vi "Mask from ROI.vi"(6 "Shrink":bool, 7 "ROI Descriptor":T1 {"Contours"."Type" items=["No Selection", "Point", "Line", "Rectangle", "Oval", "Polygon", "Free", "Annulus", "Unused2", "Unused3", "Broken Line", "Free Hand Line", "Rotated Rectangle"]}, 8 "error in (no error)":errorcluster, 9 "Out / In":bool, 11 "Image Src":T2) -> (0 "error out":errorcluster, 3 "Image Out":T2)   [LabVIEW 2014]
doc: "Recopies the Image Src into the Image Dst. You can specify if the pixels that are inside the ROI or outside the ROI are set to 0."
uses:
  <vilib>/vision/Image Controls.llb/IMAQ Image.ctl
  <vilib>/vision/NI_Vision_Development_Module.lvlib
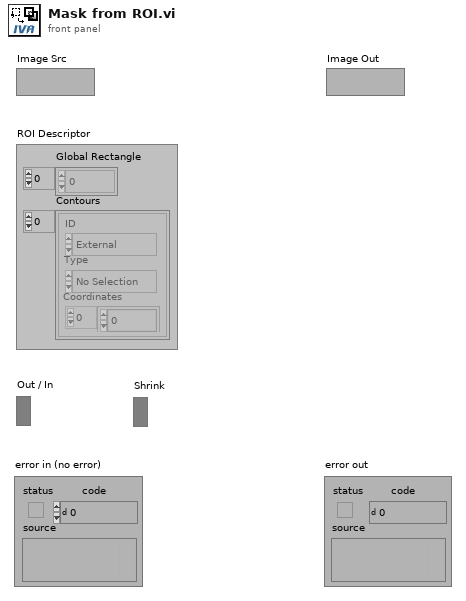
[diagram p1: front panel]
types:
  T1 = cluster{"Global Rectangle":i32[], "Contours":cluster{"ID":enum32{"External", "Internal"}, "Type":u32, "Coordinates":i32[]}[]}
  T2 = typedef "IMAQ Image.ctl" = refnum<image>
  T3 = cluster{"ID":enum32{"External", "Internal"}, "Type":u32, "Coordinates":i32[]}[]
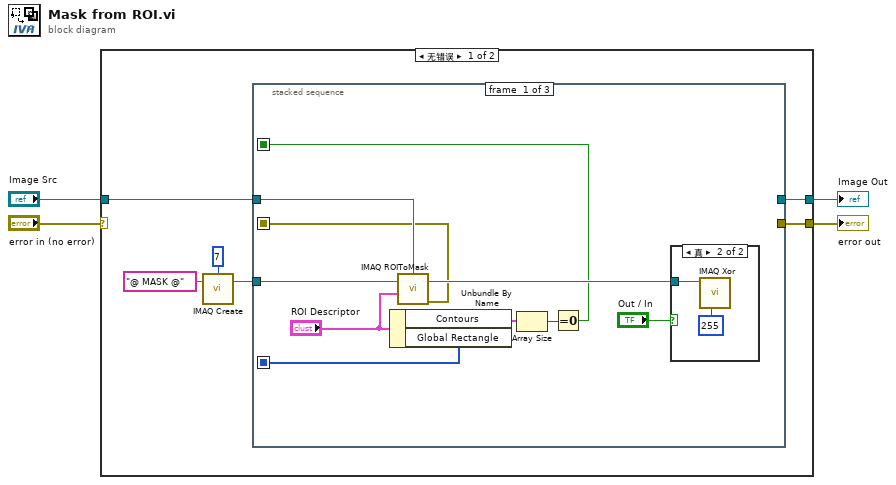
[diagram p0: block diagram]
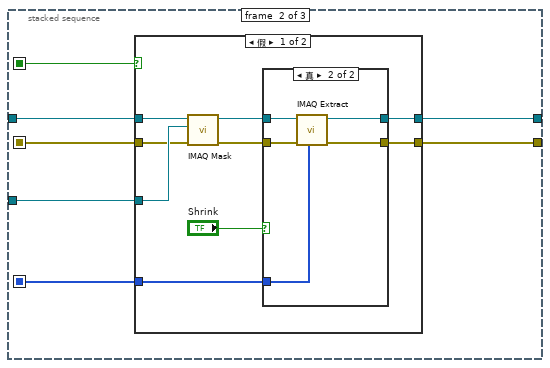
[diagram p3: hidden frame]
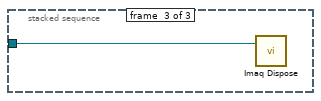
[diagram p6: hidden frame]
diagram:
  n1 = case shown="无错误" "error in (no error)" {
    selector: "error in (no error)" -> [_ w50]
    tunnel: [w8 w50] -> w4
    tunnel: "Image Src" -> [w6 w49]
    tunnel: [w5 w49] -> w2
    frame No Error {
      n2 = call "IMAQ Create"("Border Size"=7, "Image Name"="@ MASK @") -> ("New Image"=w9:T2)  [unwired: 3 in, 1 out]
      n3 = stacked-sequence {
        seq-local: [w12 _ _] -> [_ w29 _]
        seq-local: [w17 _ _] -> [_ w26 _]
        seq-local: [w11 _ _] -> [_ w24 _]
        tunnel: w6 -> [w18 w28 _]
        tunnel: w9 -> [w20 w27 w48]
        tunnel: [_ w23 _] -> w8
        tunnel: [_ w25 _] -> w5
        frame #0 {
          n4 = Unbundle By Name("ROI Descriptor") -> ("Contours"=w13:T3, "Global Rectangle"=w12:i32[])
          n5 = call "IMAQ ROIToMask"("ROI Descriptor"="ROI Descriptor", "Image"=w20, "Image Model"=w18) -> ("error out"=w11:errorcluster, "Image Out"=w19:T2)  [unwired: 3 in, 1 out]
          n6 = Array Size(array=w13) -> (size(s)=w16:i32)
          n7 = Equal To 0?(x=w16) -> (x = 0?=w17:bool)
          n8 = case shown="真" "Out / In" {
            tunnel: w19 -> [_ w22]
            frame False {
            }
            frame True {
              n9 = call "IMAQ Xor"("Constant"=255, "Image Src A"=w22) -> ()  [unwired: 8 in, 2 out]
            }
          }
        }
        frame #1 {
          n10 = case shown="假" w26 {
            tunnel: w29 -> [w38 _]
            tunnel: [w37 w47] -> w25
            tunnel: w28 -> [w36 w47]
            tunnel: w27 -> [w34 _]
            tunnel: w24 -> [w32 w46]
            tunnel: [w30 w46] -> w23
            frame False {
              n11 = call "IMAQ Mask"("error in (no error)"=w32, "Image Mask"=w34, "Image Src"=w36) -> ("error out"=w31:errorcluster, "Image Dst Out"=w35:T2)  [unwired: 2 in]
              n12 = case shown="真" "Shrink" {
                tunnel: w35 -> [w40 w45]
                tunnel: w38 -> [_ w44]
                tunnel: [w40 w43] -> w37
                tunnel: w31 -> [w39 w42]
                tunnel: [w39 w41] -> w30
                frame False {
                }
                frame True {
                  n13 = call "IMAQ Extract"("Optional Rectangle"=w44, "error in (no error)"=w42, "Image Src"=w45) -> ("error out"=w41:errorcluster, "Image Dst Out"=w43:T2)  [unwired: 7 in]
                }
              }
            }
            frame True {
            }
          }
        }
        frame #2 {
          n14 = call "Imaq Dispose"("Image"=w48) -> ()  [unwired: 5 in, 1 out]
        }
      }
    }
    frame Error {
    }
  }
  "error out" <- w4
  "Image Out" <- w2
